vi "dmm_measurement_without_teststand.vi"() -> (0 "error out":errorcluster)   [LabVIEW 2012]
panel:
  out "Reading 2":dbl format="%.2f"
  out "Reading 1":dbl format="%.2f"
  in  "Session Name":string="SampleDMM"
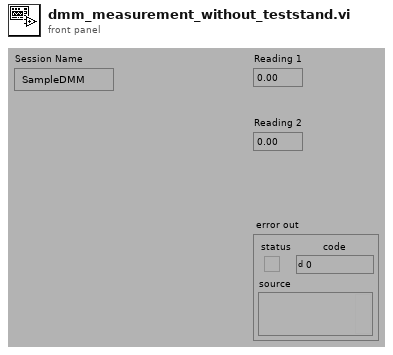
[diagram p1: front panel]
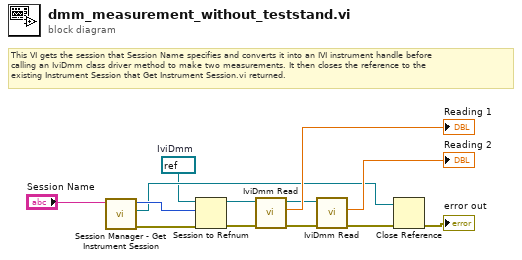
[diagram p0: block diagram]
diagram:
  w1 = refnum<k15> refnum  # IviDmm
  # "This VI gets the session that Session Name specifies and converts it into an IVI instrument handle before\ncalling an IviDmm class driver method to make two measurements. It then closes the reference to the\nexisting Instrument Session that Get Instrument Session.vi returned."
  n1 = call <vilib>:"Session Manager - Get Instrument Session.vi"("Session Name"="Session Name") -> ("error out"=w12:errorcluster, "Instrument Session"=w3:refnum<k7>, "Driver Handle"=w13:u32)  [unwired: 2 in, 6 out]
  n2 = Session to Refnum(4:w12, 6:w13, 7:w1) -> (0:w11:errorcluster, 3:w10:refnum<k15>)
  n3 = call <vilib>:"IviDmm Read.vi"("error in (no error)"=w11, "instrument handle"=w10) -> ("error out"=w7:errorcluster, "reading"=→"Reading 1":dbl, "instrument handle out"=w5:refnum<k15>)  [unwired: 1 in, 6 out]
  n4 = call <vilib>:"IviDmm Read.vi"("error in (no error)"=w7, "instrument handle"=w5) -> ("error out"=w4:errorcluster, "reading"=→"Reading 2":dbl)  [unwired: 1 in, 7 out]
  n5 = Close Reference(reference=w3, error in (no error)=w4) -> (error out=→"error out":errorcluster)
